vi "timestampISO8601String.vi"(9 "Time Stamp":timestamp format="%<%x %.3X>T", 10 "When?":enum16{"Now", "Use Input"}(ring)=enum."Use Input") -> (0 "date/timeWithSeconds":string, 1 "date/time":string, 2 "timestampString":string, 3 "timestamp":ext format="%.3f", 4 "Time(24h)":string, 5 "Date(YYYY-MM-DD)":string)   [LabVIEW 2022 SP3]
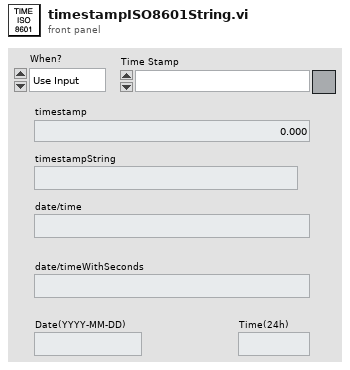
[diagram p1: front panel]
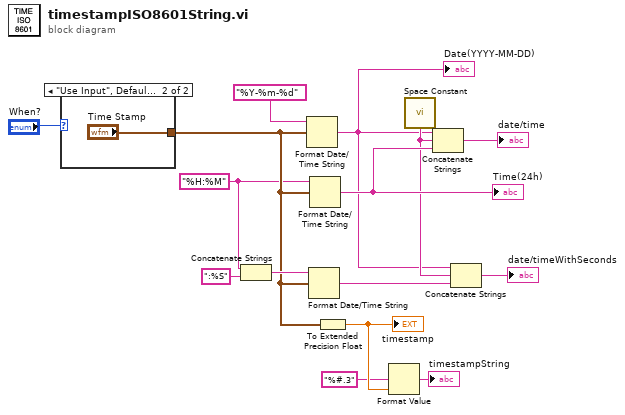
[diagram p0: block diagram]
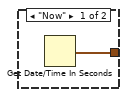
[diagram p2: hidden frame]
diagram:
  w4 = "%H:%M" ("time format string (%c)")
  n1 = case shown="\"Use Input\", Default" "When?" {
    tunnel: [w16 "Time Stamp"] -> w7
    frame "Now" {
      n2 = Get Date/Time In Seconds() -> (seconds since 1Jan1904=w16:timestamp)
    }
    frame "Use Input", Default {
    }
  }
  n3 = Concatenate Strings(w4, ":%S" ("string")) -> (w14:string)
  n4 = Format Date/Time String(time format string (%c)="%Y-%m-%d", seconds (now)=w7) -> (date/time string=w1:string)  [unwired: 1 in]
  "Date(YYYY-MM-DD)" <- w1
  n5 = Format Date/Time String(time format string (%c)=w14, seconds (now)=w7) -> (date/time string=w12:string)  [unwired: 1 in]
  n6 = Format Date/Time String(time format string (%c)=w4, seconds (now)=w7) -> (date/time string=w5:string)  [unwired: 1 in]
  "Time(24h)" <- w5
  n7 = To Extended Precision Float(1:w7) -> (0:w9:ext)
  "timestamp" <- w9
  n8 = Format Value(format string="%#.3", value (0)=w9) -> (output string=→"timestampString":string)  [unwired: 1 in]
  n9 = call <vilib>:"Space Constant.vi"() -> ("String"=w2:string)
  n10 = Concatenate Strings(w1, w2, w5) -> (→"date/time":string)
  n11 = Concatenate Strings(w1, w2, w12) -> (→"date/timeWithSeconds":string)
